vi "Merge Error.vi"(10 "Error":errorcluster, 11 "Ex Queue Actor in":refnum<class "Ex Queue Actor.lvclass">) -> (3 "Ex Queue Actor out":refnum<class "Ex Queue Actor.lvclass">)   [LabVIEW 2021, in "Ex Queue Actor.lvlib" / "Ex Queue Actor.lvclass"]
uses:
  Ex Queue Actor.lvclass
  Ex Queue Actor.lvclass/Ex Queue Actor.ctl
  Actor/Queue Actor/Queue Actor.lvclass
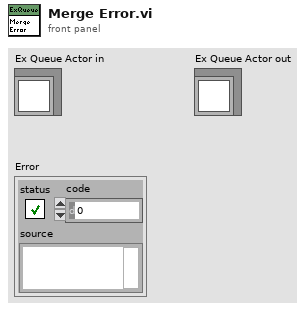
[diagram p1: front panel]
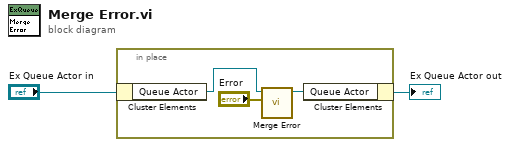
[diagram p0: block diagram]
diagram:
  n1 = in-place {
    n2 = in-place-cluster #1("Ex Queue Actor in") -> ("Queue Actor"=w5:refnum<class "Queue Actor.lvclass">)
    n3 = call-dynamic "Merge Error.vi"("Error"="Error", "Set Error in"=w5) -> ("Set Error out"=w4:refnum<class "Queue Actor.lvclass">)  [unwired: 9 in]
    n4 = in-place-cluster #1("Queue Actor"=w4) -> (→"Ex Queue Actor out":refnum<class "Ex Queue Actor.lvclass">)
  }
